vi "LIDAR Serial Read Write.vi"   [LabVIEW 2009]
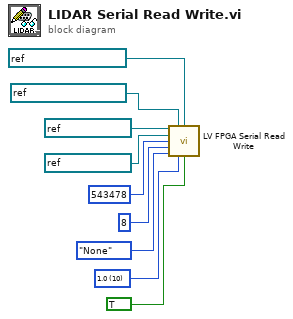
[diagram p0: block diagram]
diagram:
  w6 = u16 10 items=["1.0"=10, "1.5"=15, "2.0"=20] ("stop bits (10: 1 bit)")
  n1 = call "LV FPGA Serial Read Write.vi"("Transmit"=refnum<k21> "Port4/DIO7", "Read FIFO"=refnum<k21> "LIDAR Read FIFO", "Write FIFO"=refnum<k21> "LIDAR Write FIFO", "Receive"=refnum<k21> "Port4/DIO8", "baud rate (9600)"=u32 543478, "data bits (8)"=8, "parity (0:none)"=enum16{"None", "Odd", "Even", "Mark", "Space"}."None", "stop bits (10: 1 bit)"=w6, "Invert Polarity?"=TRUE) -> ()  [unwired: 7 in]
